vi "dR.vi"(10 "DR/R parameter":T2, 11 "数组":u8[][][](array[numeric])) -> (3 "Image Dst Out":T1)   [LabVIEW 2011]
uses:
  <vilib>/vision/Image Controls.llb/IMAQ Image.ctl
  <vilib>/vision/NI_Vision_Development_Module.lvlib
panel:
  out "数组 2":bool[](array[boolean])
  out "Image":T1(plugin-control)
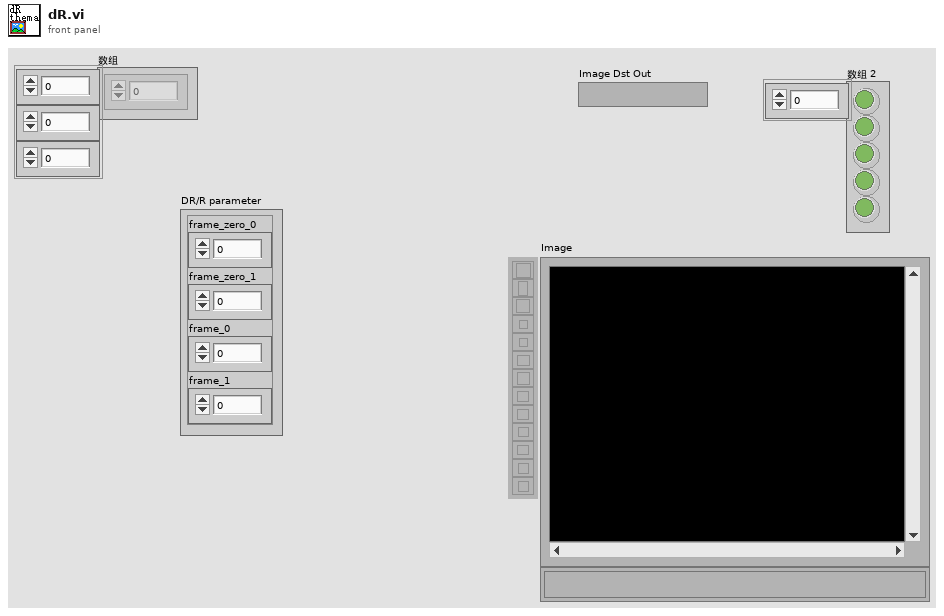
[diagram p1: front panel]
types:
  T1 = typedef "IMAQ Image.ctl" = refnum<image>
  T2 = cluster{"frame_zero_0":i32, "frame_zero_1":i32, "frame_0":i32, "frame_1":i32}
  T3 = typedef "Image Type" = u32
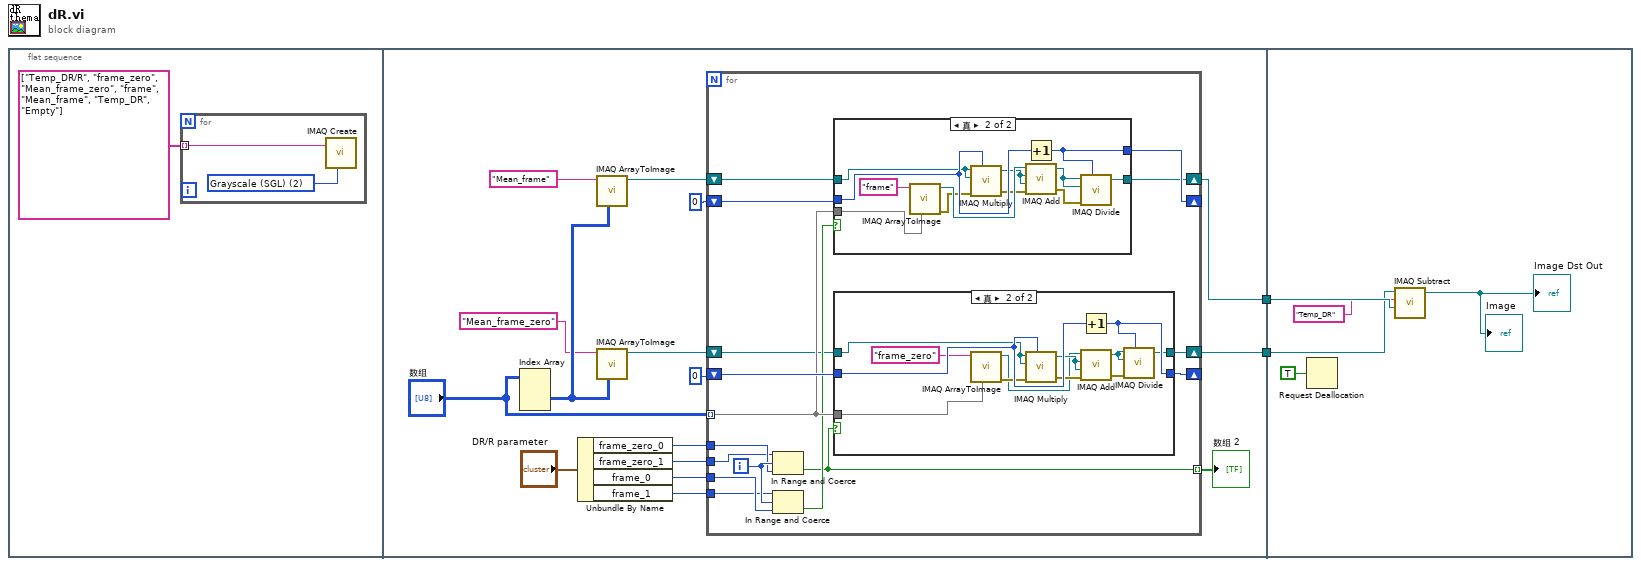
[diagram p0: block diagram]
diagram:
  n1 = flat-sequence {
    tunnel: [w13] -> w2
    tunnel: [w7] -> w1
    tunnel: w2 -> [w68]
    tunnel: w1 -> [w69]
    frame #0 {
      n2 = for {
        tunnel: string[] ["Temp_DR/R", "frame_zero", "Mean_frame_zero", "frame", "Mean_frame", "Temp_DR", "Empty"] ("添加的数组") -> [w4] mode=indexing
        w5 = T3 2 items=["Grayscale (U8)", "Grayscale (I16)", "Grayscale (SGL)", "Complex (CSG)", "RGB (U32)", "HSL (U32)", "RGB (U64)", "Grayscale (U16)"] ("Image Type")
        n3 = call "IMAQ Create"("Image Name"=w4, "Image Type"=w5) -> ()  [unwired: 3 in, 2 out]
      }
    }
    frame #1 {
      n4 = Index Array(array="数组") -> (element=w12:u8[][])  [unwired: 3 in]
      n5 = Unbundle By Name("DR/R parameter") -> ("frame_zero_0"=w20:i32, "frame_zero_1"=w19:i32, "frame_0"=w17:i32, "frame_1"=w16:i32)
      n6 = call "IMAQ ArrayToImage"("Image Pixels (Float)"=w12, "Image"="Mean_frame" ("Image Name")) -> ("Image Out"=w9:T1)  [unwired: 8 in, 1 out]
      n7 = call "IMAQ ArrayToImage"("Image Pixels (Float)"=w12, "Image"="Mean_frame_zero" ("Image Name")) -> ("Image Out"=w8:T1)  [unwired: 8 in, 1 out]
      n8 = for {
        tunnel: "数组" -> [w34] mode=indexing
        tunnel: w20 -> [w29]
        tunnel: w19 -> [w28]
        shift-right: [w36] -> _
        shift-left: 0 -> [w37]
        tunnel: w17 -> [w27]
        tunnel: w16 -> [w26]
        shift-right: [w32] -> _
        shift-left: 0 -> [w33]
        tunnel: [w30] -> w14 mode=indexing
        shift-right: [w25] -> w13
        shift-left: w8 -> [w24]
        shift-right: [w23] -> w7
        shift-left: w9 -> [w22]
        i -> [w35]
        n9 = In Range and Coerce(upper limit=w28, x=w35, lower limit=w29) -> (In Range?=w30:bool)  [unwired: 1 out]
        n10 = In Range and Coerce(upper limit=w26, x=w35, lower limit=w27) -> (In Range?=w31:bool)  [unwired: 1 out]
        n11 = case shown="真" w31 {
          tunnel: w34 -> [_ w51]
          tunnel: w33 -> [w39 w49]
          tunnel: [w39 w43] -> w32
          tunnel: [w38 w41] -> w23
          tunnel: w22 -> [w38 w40]
          frame False {
          }
          frame True {
            n12 = call "IMAQ ArrayToImage"("Image Pixels (Float)"=w51, "Image"="frame" ("Image Name")) -> ("error out"=w44:errorcluster, "Image Out"=w48:T1)  [unwired: 8 in]
            n13 = call "IMAQ Multiply"("Image Src A"=w40, "Constant"=w49, "Image Dst"=w40, "error in (no error)"=w44) -> ("Image Dst Out"=w47:T1, "error out"=w45:errorcluster)  [unwired: 3 in]
            n14 = Increment(x=w49) -> (x+1=w43:i32)
            n15 = call "IMAQ Add"("Image Src A"=w48, "Image Dst"=w47, "Image Src B"=w47, "error in (no error)"=w45) -> ("Image Dst Out"=w42:T1, "error out"=w46:errorcluster)  [unwired: 3 in]
            n16 = call "IMAQ Divide"("Image Src A"=w42, "Constant"=w43, "Image Dst"=w42, "error in (no error)"=w46) -> ("Image Dst Out"=w41:T1)  [unwired: 3 in, 1 out]
          }
        }
        n17 = case shown="真" w30 {
          tunnel: w34 -> [_ w65]
          tunnel: w37 -> [w53 w64]
          tunnel: [w53 w60] -> w36
          tunnel: [w52 w55] -> w25
          tunnel: w24 -> [w52 w54]
          frame False {
          }
          frame True {
            n18 = call "IMAQ ArrayToImage"("Image Pixels (Float)"=w65, "Image"="frame_zero" ("Image Name")) -> ("error out"=w61:errorcluster, "Image Out"=w56:T1)  [unwired: 8 in]
            n19 = call "IMAQ Multiply"("Image Src A"=w54, "Constant"=w64, "Image Dst"=w54, "error in (no error)"=w61) -> ("Image Dst Out"=w57:T1, "error out"=w62:errorcluster)  [unwired: 3 in]
            n20 = Increment(x=w64) -> (x+1=w60:i32)
            n21 = call "IMAQ Add"("Image Src A"=w56, "Image Dst"=w57, "Image Src B"=w57, "error in (no error)"=w62) -> ("Image Dst Out"=w58:T1, "error out"=w63:errorcluster)  [unwired: 3 in]
            n22 = call "IMAQ Divide"("Image Src A"=w58, "Constant"=w60, "Image Dst"=w58, "error in (no error)"=w63) -> ("Image Dst Out"=w55:T1)  [unwired: 3 in, 1 out]
          }
        }
      }
      "数组 2" <- w14
    }
    frame #2 {
      n23 = Request Deallocation(TRUE ("标志")) -> ()
      n24 = call "IMAQ Subtract"("Image Src A"=w68, "Image Dst"="Temp_DR" ("Image Name"), "Image Src B"=w69) -> ("Image Dst Out"=→"Image Dst Out" →"Image":T1)  [unwired: 4 in, 1 out]
    }
  }
